vi "Main.vi"() -> ()   [LabVIEW 2020]
uses:
  <vilib>/Utility/file.llb/Read Delimited Spreadsheet (string).vi
  <vilib>/Utility/file.llb/Write Delimited Spreadsheet (string).vi
panel:
  out "Size":i32
  in  "Configs":i32(listbox)
  in  "Config File":string="CFG-VALGET - 06 8B 90 02 01 00 80 04 09 00 A4 40 00 90 D0 03 0A 00 A4 40 00 20 A1 07 0B 00 A4 40 00 90 D0 03 0C 00 A4 40 00 24 F4 00 0D 00 A4 40 E0 87 F4 02 10 00 A4 40 00 B0 71 0B 01 00 A5 40 01 00 00 00 05 00 A5 40 FF FF FF 1F 06 00 A5 40 FF FF FF FF 07 00 A5 40 FF FF FF FF 08 00 A5 40 FF FF FF FF 09 00 A5 40 FF FF FF FF 01 00 A6 40 00 00 00 00 34 00 C6 40 0F 00 00 00 14 00 D0 40 3C 00 00 00 15 00 D0 40 30 00 00 00 08 00 DE 40 00 00 00 00 2A 00 05 50 00 00 00 00 00 00 00 00 2B 00 05 50 00 00 00 00 00 00 24 40 62 00 11 50 00 00 00 40 A6 54 58 41 63 00 11 50 88 6D 74 96 1D A4 72 40 06 00 36 50 C8 2B 07 00 00 00 00 00 0D 00 65 50 75 2D 62 6C 6F 78 20 41 0E 00 65 50 47 20 2D 20 77 77 77 2E 0F 00 65 50 75 2D 62 6C 6F 78 2E 63 10 00 65 50 6F 6D 00 00 00 00 00 00 11 00 65 50 75 2D 62 6C 6F 78 20 47 12 00 65 50 4E 53 53 20 72 65 63 65 13 00 65 50 69 76 65 72 00 00 00 00 14 00 65 50 00 00 00 00 00 00 00 00 15 00 65 50 00 00 00 00 00 00 00 00 16 00 65 50 00 00 00 00 00 00 00 00 17 00 65 50 00 00 00 00 00 00 00 00 18 00 65 50 00 00 00 00 00 00 00 00 26 00 A3 50 20 40 00 00 54 00 00 00 49 00 A3 50 5A 45 44 2D 46 39 50 00 03 00 A5 50 4D 77 35 A3 ED 01 00 00 07 00 C6 50 00 00 00 00 00 00 00 00 0B 00 C6 50 00 00 00 00 00 00 00 00 0F 00 C6 50 00 00 00 00 00 00 00 00 13 00 C6 50 00 00 00 00 00 00 00 00 17 00 C6 50 00 00 00 00 00 00 00 00 1B 00 C6 50 00 00 00 00 00 00 00 00 1F 00 C6 50 00 00 00 00 00 00 00 00 23 00 C6 50 00 00 00 00 00 00 00 00 27 00 C6 50 00 00 00 00 00 00 00 00 2B 00 C6 50 00 00 00 00 00 00 00 00 2F 00 C6 50 00 00 00 00 00 00 00 00 33 00 C6 50 00 00 00 00 00 00 00 00 04 00 C7 50 4E 6F 74 69 63 65 3A 20 05 00 C7 50 6E 6F 20 64 61 74 61 20 06 00 C7 50 73 61 76 65 64 21 00 00 07 00 C7 50 00 00 00 00 00 00 00 00 02 00 F6 50 00 00 00 00 00 00 00 00 03 00 F6 50 00 00 00 00 00 00 00 00 04 00 F6 50 00 00 00 00 00 00 00 00 05 00 F6 50 00 00 00 00 00 00 00 00 06 00 F6 50 00 00 00 00 00 00 00 00 07 00 F6 50 00 00 00 00 00 00 00 00 08 00 F6 50 00 00 00 00 00 00 00 00\n"
  in  "file path (dialog if empty)":path
  # "Class\nID\nLength lo\nLength hi\nversion\nlayers\nreserved1\nreserved 2\ncfgData\n  |\n  |\n \\/"
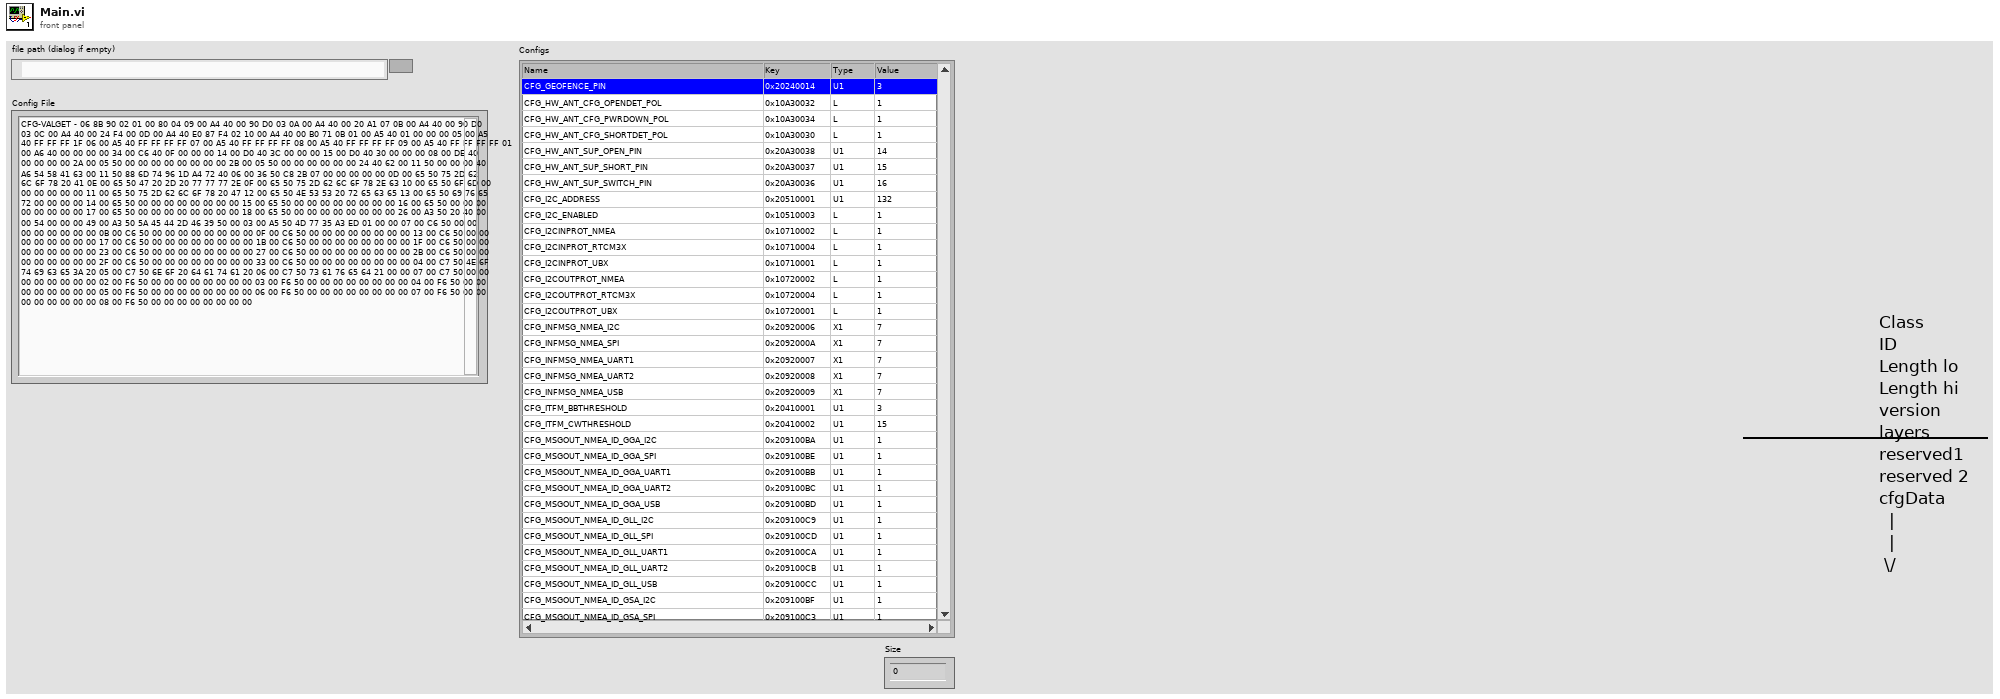
[diagram p1: front panel]
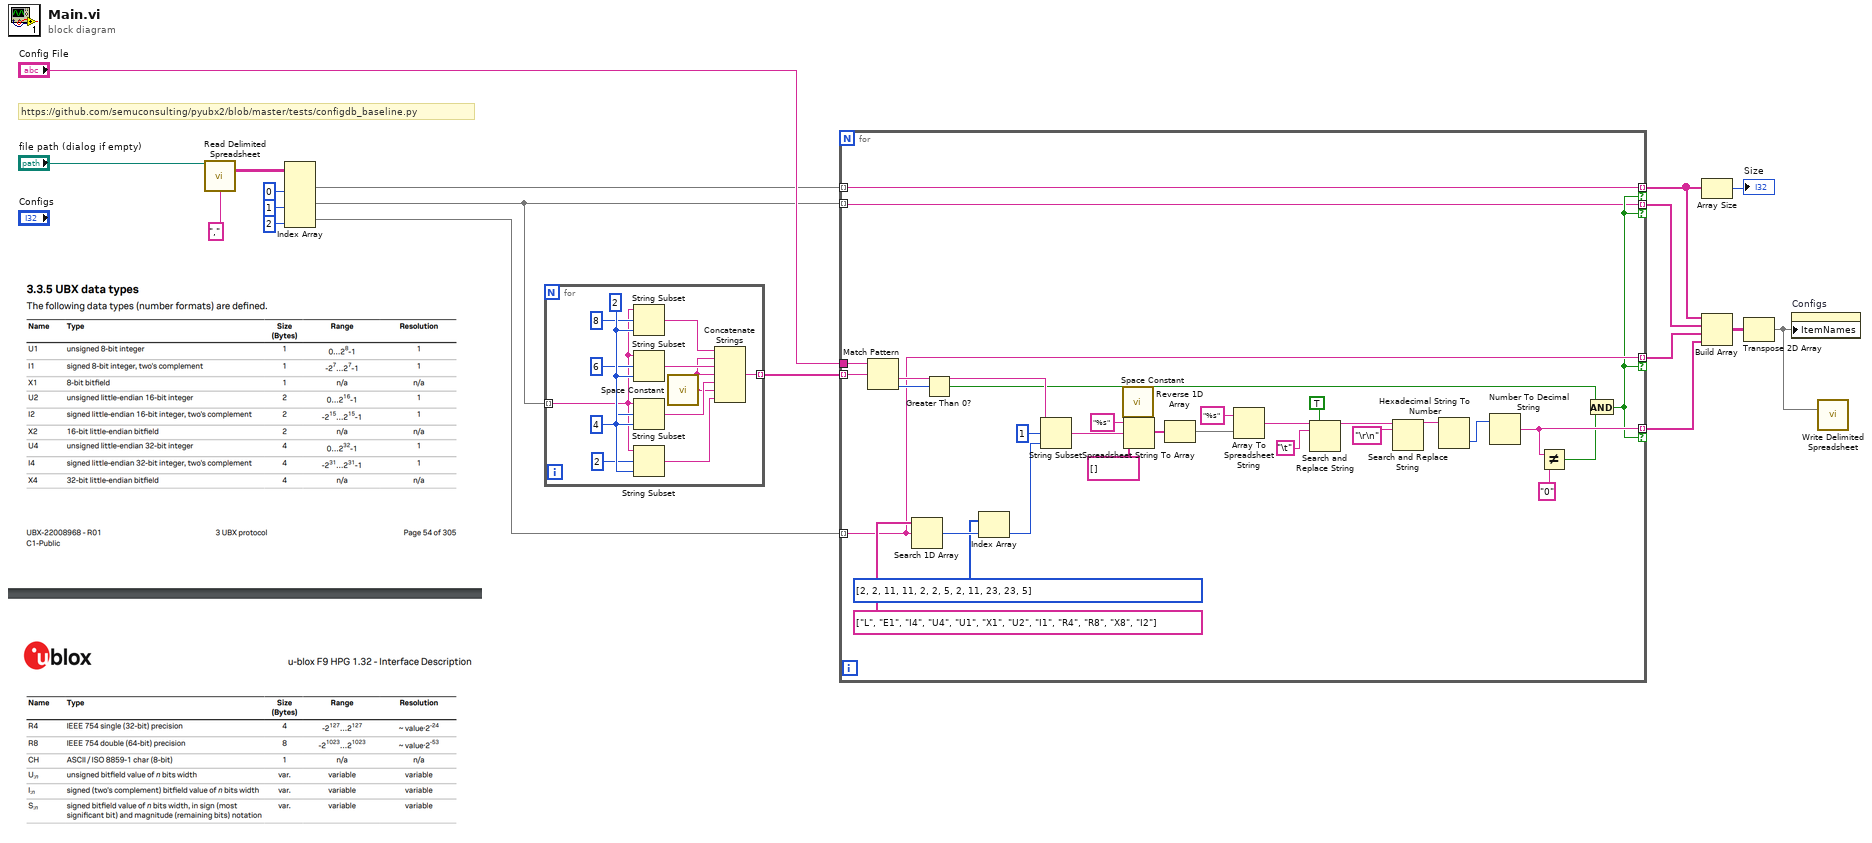
[diagram p0: block diagram]
diagram:
  # "https://github.com/semuconsulting/pyubx2/blob/master/tests/configdb_baseline.py"
  n1 = call-poly <vilib>:"Read Delimited Spreadsheet.vi"("file path (dialog if empty)"="file path (dialog if empty)", "delimiter (\\t)"="," ("delimiter (\\t)")) -> ("all rows"=w3:string[][])  [unwired: 8 in, 5 out]
  n2 = Index Array(array=w3, index (col) #1=0 ("disabled index (col)"), index (col) #2=1 ("index (col)"), index (col) #3=2 ("index (col)")) -> (element #1=w9:string[], element #2=w8:string[], element #3=w7:string[])  [unwired: 3 in]
  n3 = for {
    tunnel: w8 -> [w20] mode=indexing
    tunnel: [w21] -> w16 mode=indexing
    w30 = 2 ("length (rest)")
    n4 = String Subset(string=w20, offset (0)=8, length (rest)=w30) -> (substring=w26:string)
    n5 = String Subset(string=w20, offset (0)=6, length (rest)=w30) -> (substring=w25:string)
    n6 = String Subset(string=w20, offset (0)=4, length (rest)=w30) -> (substring=w24:string)
    n7 = String Subset(string=w20, offset (0)=2, length (rest)=w30) -> (substring=w23:string)
    n8 = call <vilib>:"Space Constant.vi"() -> ("String"=w22:string)
    n9 = Concatenate Strings(w26, w22, w25, w22, w24, w22, w23) -> (w21:string)
  }
  n10 = for {
    tunnel: "Config File" -> [w61]
    tunnel: w16 -> [w52] mode=indexing
    tunnel: w9 -> [w59] mode=indexing
    tunnel: [w59] -> w1 mode=indexing if=w33
    tunnel: w7 -> [w51] mode=indexing
    tunnel: [w37] -> w12 mode=indexing if=w33
    tunnel: [w51] -> w14 mode=indexing if=w33
    tunnel: w8 -> [w32] mode=indexing
    tunnel: [w32] -> w13 mode=indexing if=w33
    n11 = Match Pattern(string=w61, regular expression=w52) -> (after substring=w55:string, offset past match=w60:i32)  [unwired: 1 in, 2 out]
    n12 = Search 1D Array(1D array=string[] ["L", "E1", "I4", "U4", "U1", "X1", "U2", "I1", "R4", "R8", "X8", "I2"] ("Output Array"), element=w51) -> (index of element=w57:i32)  [unwired: 1 in]
    n13 = Greater Than 0?(x=w60) -> (x > 0?=w35:bool)
    n14 = Index Array(array=i32[] [2, 2, 11, 11, 2, 2, 5, 2, 11, 23, 23, 5], index=w57) -> (element=w54:i32)
    n15 = String Subset(string=w55, offset (0)=1, length (rest)=w54) -> (substring=w50:string)
    n16 = call <vilib>:"Space Constant.vi"() -> ("String"=w49:string)
    n17 = Spreadsheet String To Array(delimiter (Tab)=w49, format string="%s", spreadsheet string=w50, array type (2D Dbl)=string[] []) -> (array=w47:string[])
    n18 = Reverse 1D Array(array=w47) -> (reversed array=w45:string[])
    n19 = Array To Spreadsheet String(array=w45, 3:"%s" ("format string")) -> (spreadsheet string=w43:string)  [unwired: 1 in]
    n20 = Search and Replace String(replace all?=TRUE ("replace all? (F)"), input string=w43, search string="\t") -> (result string=w40:string)  [unwired: 5 in, 3 out]
    n21 = Search and Replace String(input string=w40, search string="\r\n" ("format string")) -> (result string=w31:string)  [unwired: 6 in, 3 out]
    n22 = Hexadecimal String To Number(string=w31) -> (number=w38:u32)  [unwired: 2 in, 1 out]
    n23 = Number To Decimal String(number=w38) -> (decimal integer string=w37:string)  [unwired: 1 in]
    n24 = Not Equal?(x=w37, y="0") -> (x != y?=w34:bool)
    n25 = And(x=w35, y=w34) -> (x .and. y?=w33:bool)
  }
  n26 = Array Size(array=w1) -> (size(s)=→"Size":i32)
  n27 = Build Array(w1, w13, w14, w12) -> (w11:string[][])
  n28 = Transpose 2D Array(2D array=w11) -> (transposed array=w10:string[][])
  n29 = property on="Configs" class="MCListbox (strict)"("ItemNames"=w10) -> ()  [unwired: 2 in, 2 out]
  n30 = call-poly <vilib>:"Write Delimited Spreadsheet.vi"("2D data"=w10) -> ()  [unwired: 13 in, 2 out]
